vi "Modified File Dialog.vi"(0 "Start Path":path=path "" caption="start path", 1 "Prompt":string, 3 "Button Label":string caption="button label", 7 "Suggested Filename":string, 11 "error in (no error)":errorcluster, 12 "Pattern":string, 14 "Pattern Label":string) -> (4 "Selected Path":path, 8 "File exists":bool, 10 "Cancelled":bool, 15 "error out":errorcluster)   [LabVIEW 2021, in "Files.lvlib"]
uses:
  Files.lvlib
  GUI/GUI.lvlib
panel:
  # "see the License on the block diagram (Ctrl+E or Window:Show Block Diagram)"
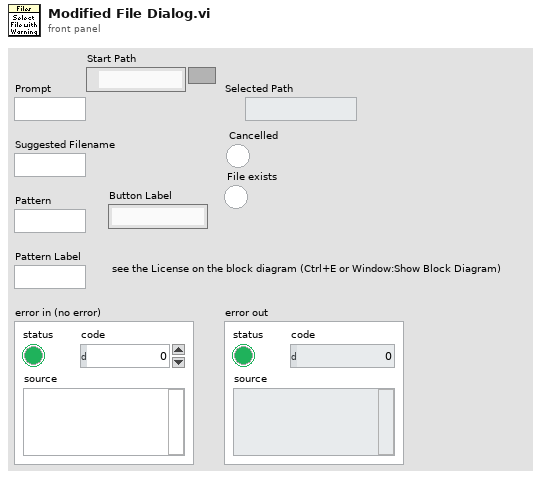
[diagram p1: front panel]
types:
  T1 = typedef "Fits.lvlib/3-Button Dialog Output.ctl" = enum16{"Window Close", "Button 1", "Button 2", "Button 3"}
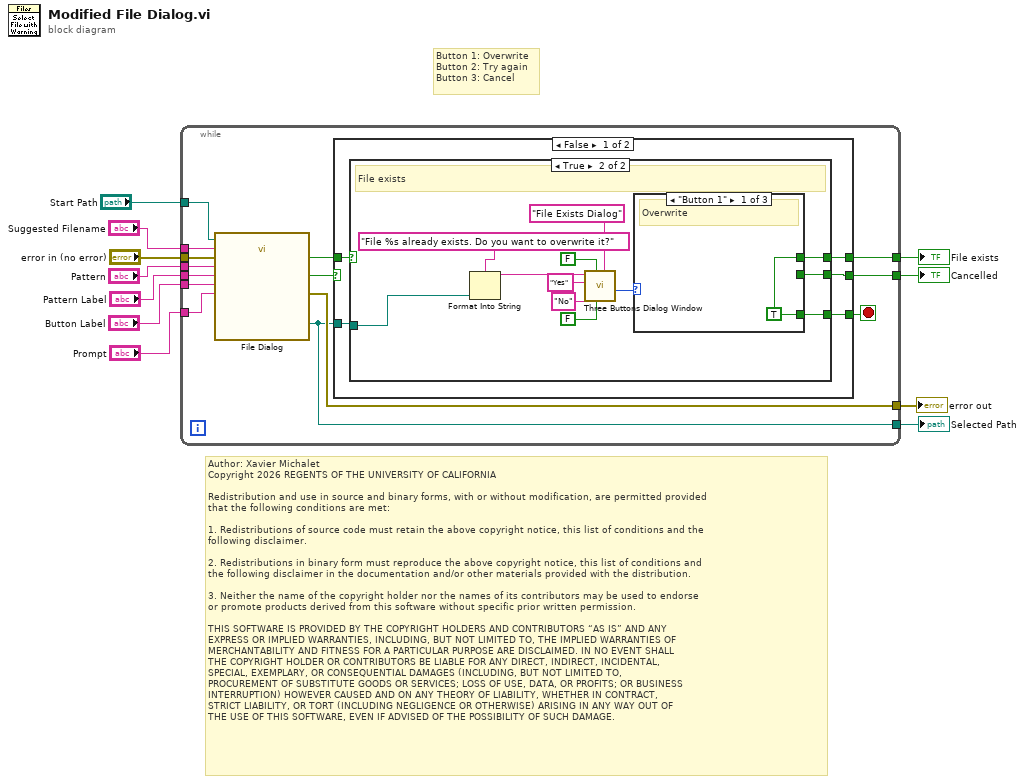
[diagram p0: block diagram]
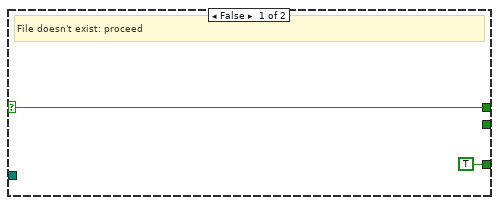
[diagram p2: hidden frame]
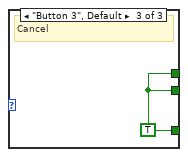
[diagram p4: hidden frame]
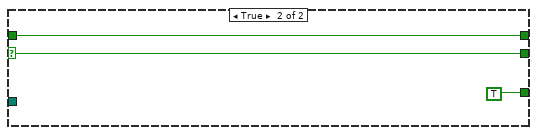
[diagram p5: hidden frame]
diagram:
  # "Author: Xavier Michalet\nCopyright 2026 REGENTS OF THE UNIVERSITY OF CALIFORNIA\n\nRedistribution and use in source and binary forms, with or without modification, are permitted provided\nthat the following conditions are met:\n\n1. Redistributions of source code must retain the above copyright notice, this list of conditions and the\nfollowing disclaimer.\n\n2. Redistributions in binary form must reproduce the above copyright notice, this list of conditions and\nthe following disclaimer in the documentation and/or other materials provided with the distribution.\n\n3. Neither the name of the copyright holder nor the names of its contributors may be used to endorse \nor promote products derived from this software without specific prior written permission.\n\nTHIS SOFTWARE IS PROVIDED BY THE COPYRIGHT HOLDERS AND CONTRIBUTORS “AS IS” AND ANY \nEXPRESS OR IMPLIED WARRANTIES, INCLUDING, BUT NOT LIMITED TO, THE IMPLIED WARRANTIES OF\nMERCHANTABILITY AND FITNESS FOR A PARTICULAR PURPOSE ARE DISCLAIMED. IN NO EVENT SHALL\nTHE COPYRIGHT HOLDER OR CONTRIBUTORS BE LIABLE FOR ANY DIRECT, INDIRECT, INCIDENTAL, \nSPECIAL, EXEMPLARY, OR CONSEQUENTIAL DAMAGES (INCLUDING, BUT NOT LIMITED TO, \nPROCUREMENT OF SUBSTITUTE GOODS OR SERVICES; LOSS OF USE, DATA, OR PROFITS; OR BUSINESS\nINTERRUPTION) HOWEVER CAUSED AND ON ANY THEORY OF LIABILITY, WHETHER IN CONTRACT, \nSTRICT LIABILITY, OR TORT (INCLUDING NEGLIGENCE OR OTHERWISE) ARISING IN ANY WAY OUT OF\nTHE USE OF THIS SOFTWARE, EVEN IF ADVISED OF THE POSSIBILITY OF SUCH DAMAGE."
  # "Button 1: Overwrite\nButton 2: Try again\nButton 3: Cancel"
  n1 = while {
    tunnel: "Suggested Filename" -> [w25]
    tunnel: "Prompt" -> [w23]
    tunnel: "Pattern" -> [w22]
    tunnel: "Pattern Label" -> [w21]
    tunnel: [w18] -> w6
    tunnel: "error in (no error)" -> [w24]
    tunnel: [w20] -> w5
    tunnel: [w16] -> w4
    tunnel: [w15] -> w3
    tunnel: "Start Path" -> [w13]
    tunnel: "Button Label" -> [w12]
    stop <- w17 stop-if-true
    n2 = call "File Dialog"("start path"=w13, "prompt"=w23, "button label"=w12, "default name"=w25, "error in"=w24, "pattern (all files)"=w22, "pattern label"=w21) -> ("selected path"=w18:path, "exists"=w19:bool, "cancelled"=w14:bool, "error out"=w20:errorcluster)  [unwired: 5 in]
    n3 = case shown="False" w14 {
      selector: w14 -> [_ w49]
      tunnel: w19 -> [w30 w48]
      tunnel: w18 -> [w29 _]
      tunnel: [w28 TRUE] -> w17
      tunnel: [w27 w48] -> w16
      tunnel: [w26 w49] -> w15
      frame False {
        n4 = case shown="True" w30 {
          selector: w30 -> [w31 _]
          tunnel: w29 -> [_ w40]
          tunnel: [TRUE w39] -> w28
          tunnel: [w31 w38] -> w27
          tunnel: [_ w37] -> w26
          frame False {
            # "File doesn't exist: proceed"
          }
          frame True {
            # "File exists"
            n5 = Format Into String(format string="File %s already exists. Do you want to overwrite it?", w40) -> (resulting string=w42:string)  [unwired: 2 in, 1 out]
            n6 = call "Three Buttons Dialog Window.vi"("Window Title"="File Exists Dialog", "ESC =  Button 3 (T)"=FALSE, "Return =  Button 1 (T)"=FALSE, "Button 2 Text"="No", "Button 1 Text (OK)"="Yes" ("T button name (\"OK\")"), "Message"=w42) -> ("3-button Dialog Output"=w43:T1)  [unwired: 5 in]
            n7 = case shown="\"Button 1\"" w43 {
              tunnel: [w45 _ w46] -> w39
              tunnel: [w45 _ w46] -> w38
              tunnel: [_ _ w46] -> w37
              frame "Button 1" {
                w45 = TRUE
                # "Overwrite"
              }
              frame "Button 2" {
                # "Try again"
              }
              frame "Button 3", Default {
                w46 = TRUE
                # "Cancel"
              }
            }
          }
        }
      }
      frame True {
      }
    }
  }
  "error out" <- w5
  "Selected Path" <- w6
  "File exists" <- w4
  "Cancelled" <- w3
